vi "例程34-基于持续时间的信号发生器VI的使用.vi"() -> ()   [LabVIEW 2016]
uses:
  <vilib>/Analysis/NI_AALPro.lvlib
panel:
  out "波形图":dbl[](graph)
  out "error":i32 caption="错误"
  out "phase out":dbl caption="相位输出" format="%0.2e"
  out "sample rate":dbl=1.0 caption="采样率" format="%0.2f"
  out "signal":dbl[](array[numeric]) caption="信号"
  in  "square wave duty cycle (%)":dbl=50.0 caption="方波占空比(%)" format="%0.2f"
  in  "phase in":dbl caption="相位输入" format="%0.2f"
  in  "dc offset":dbl caption="直流偏移量" format="%0.2f"
  in  "amplitude":dbl=1.0 caption="幅值" format="%0.2f"
  in  "frequency":dbl=10.0 caption="频率" format="%0.2f"
  in  "# of samples":i32=100 caption="采样点数"
  in  "reset phase":bool=TRUE caption="重置相位"
  in  "duration":dbl=1.0 caption="持续时间" format="%0.2f"
  in  "signal type":T1(ring) caption="信号类型"
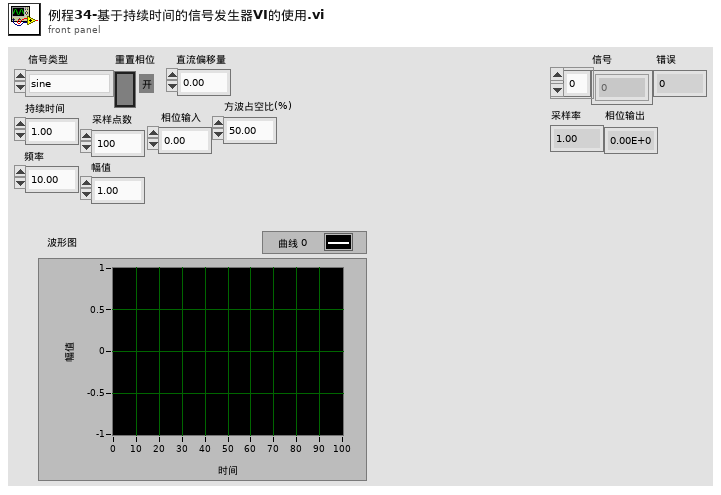
[diagram p1: front panel]
types:
  T1 = enum16{"sine", "cosine", "triangle", "square", "sawtooth", "increasing ramp", "decreasing ramp"}
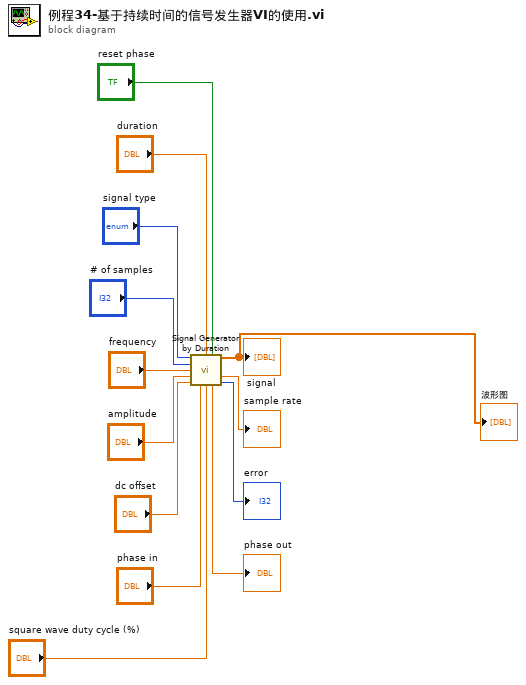
[diagram p0: block diagram]
diagram:
  n1 = call <vilib>:"Signal Generator by Duration.vi"("signal type"="signal type", "duration"="duration", "reset phase"="reset phase", "# of samples"="# of samples", "frequency"="frequency", "amplitude"="amplitude", "dc offset"="dc offset", "phase in"="phase in", "square wave duty cycle (%)"="square wave duty cycle (%)") -> ("signal"=→"signal" →"波形图":dbl[], "sample rate"=→"sample rate":dbl, "phase out"=→"phase out":dbl, "error"=→"error":i32)  [unwired: 3 in]
